vi "Set_Gain_DHPCA-100.vi"(3 "error in":errorcluster, 4 "Status":i32, 5 "Gain  [V/A]":T1(ring), 6 "index":i32) -> (0 "error out":errorcluster, 1 "Status_out":i32, 2 "index_out":i32)   [LabVIEW 2010, in "FEMTO_LUCI-10.lvlib"]
uses:
  <userlib>/FEMTO/FEMTO_LUCI-10.lvlib
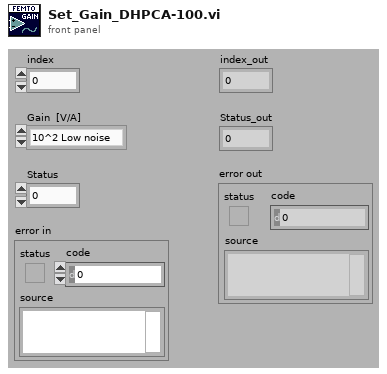
[diagram p1: front panel]
types:
  T1 = enum16{"10^2 Low noise", "10^3 Low noise", "10^4 Low noise", "10^5 Low noise", "10^6 Low noise", "10^7 Low noise", "10^3 High speed", "10^4 High speed", "10^5 High speed", "10^6 High speed", "10^7 High speed", "10^8 High speed"}
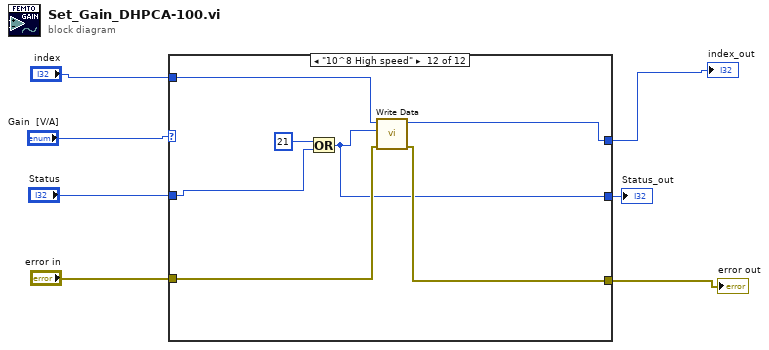
[diagram p0: block diagram]
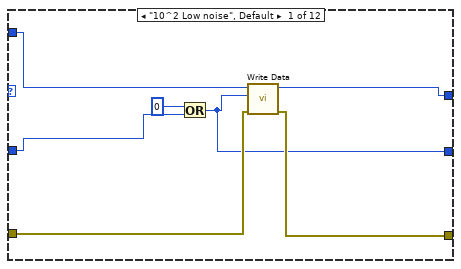
[diagram p2: hidden frame]
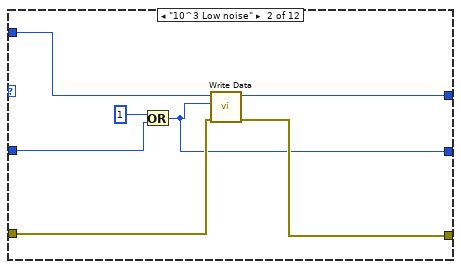
[diagram p3: hidden frame]
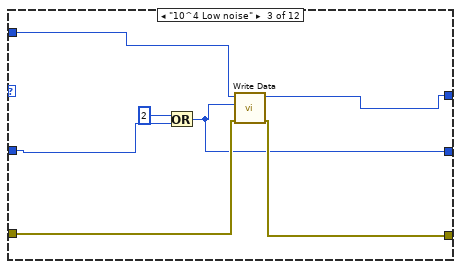
[diagram p4: hidden frame]
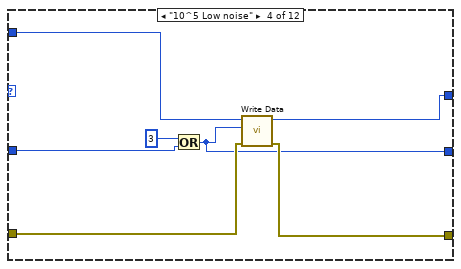
[diagram p5: hidden frame]
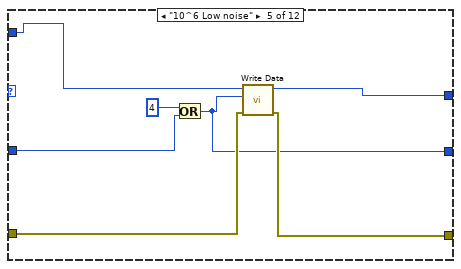
[diagram p6: hidden frame]
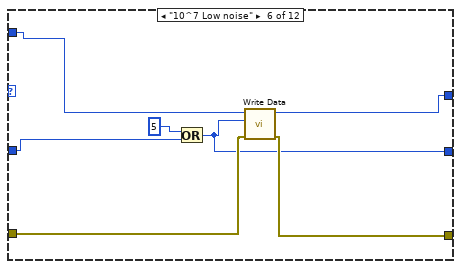
[diagram p7: hidden frame]
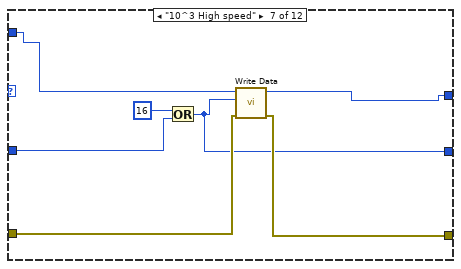
[diagram p8: hidden frame]
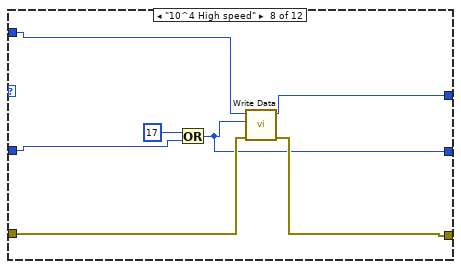
[diagram p9: hidden frame]
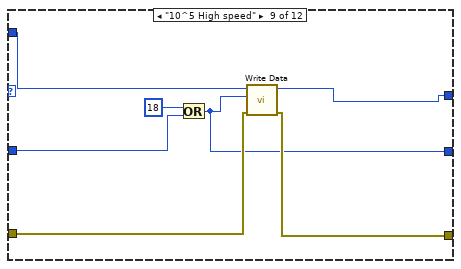
[diagram p10: hidden frame]
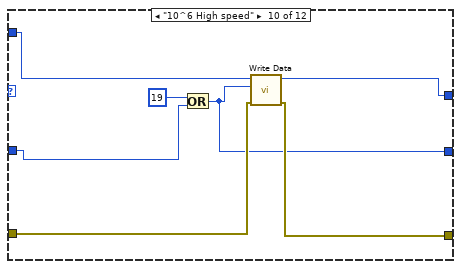
[diagram p11: hidden frame]
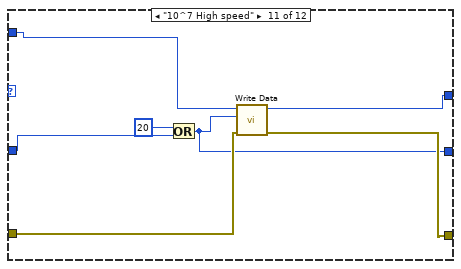
[diagram p12: hidden frame]
diagram:
  n1 = case shown="\"10^8 High speed\"" "Gain  [V/A]" {
    tunnel: "index" -> [w12 w21 w26 w33 w41 w48 w55 w61 w68 w76 w82 w89]
    tunnel: [w11 w20 w25 w32 w40 w47 w54 w62 w69 w75 w83 w88] -> w2
    tunnel: "error in" -> [w9 w19 w23 w30 w38 w45 w52 w60 w66 w73 w80 w86]
    tunnel: [w10 w18 w24 w31 w39 w46 w53 w59 w67 w74 w79 w87] -> w4
    tunnel: "Status" -> [w13 w17 w27 w34 w37 w44 w51 w58 w65 w72 w81 w90]
    tunnel: [w8 w15 w22 w29 w36 w43 w50 w57 w64 w71 w78 w85] -> w7
    frame "10^2 Low noise", Default {
      n2 = Or(x=0 ("data_low"), y=w13) -> (x .or. y?=w8:i32)
      n3 = call <userlib>:"Write Data.vi"("error in (no error)"=w9, "data_low"=w8, "index"=w12) -> ("error out"=w10:errorcluster, "index_out"=w11:i32)  [unwired: 1 in, 6 out]
    }
    frame "10^3 Low noise" {
      n4 = Or(x=1 ("data_low"), y=w17) -> (x .or. y?=w15:i32)
      n5 = call <userlib>:"Write Data.vi"("error in (no error)"=w19, "data_low"=w15, "index"=w21) -> ("error out"=w18:errorcluster, "index_out"=w20:i32)  [unwired: 1 in, 6 out]
    }
    frame "10^4 Low noise" {
      n6 = Or(x=2 ("data_low"), y=w27) -> (x .or. y?=w22:i32)
      n7 = call <userlib>:"Write Data.vi"("error in (no error)"=w23, "data_low"=w22, "index"=w26) -> ("error out"=w24:errorcluster, "index_out"=w25:i32)  [unwired: 1 in, 6 out]
    }
    frame "10^5 Low noise" {
      n8 = Or(x=3 ("data_low"), y=w34) -> (x .or. y?=w29:i32)
      n9 = call <userlib>:"Write Data.vi"("error in (no error)"=w30, "data_low"=w29, "index"=w33) -> ("error out"=w31:errorcluster, "index_out"=w32:i32)  [unwired: 1 in, 6 out]
    }
    frame "10^6 Low noise" {
      n10 = Or(x=4 ("data_low"), y=w37) -> (x .or. y?=w36:i32)
      n11 = call <userlib>:"Write Data.vi"("error in (no error)"=w38, "data_low"=w36, "index"=w41) -> ("error out"=w39:errorcluster, "index_out"=w40:i32)  [unwired: 1 in, 6 out]
    }
    frame "10^7 Low noise" {
      n12 = Or(x=5 ("data_low"), y=w44) -> (x .or. y?=w43:i32)
      n13 = call <userlib>:"Write Data.vi"("error in (no error)"=w45, "data_low"=w43, "index"=w48) -> ("error out"=w46:errorcluster, "index_out"=w47:i32)  [unwired: 1 in, 6 out]
    }
    frame "10^3 High speed" {
      n14 = Or(x=16 ("data_low"), y=w51) -> (x .or. y?=w50:i32)
      n15 = call <userlib>:"Write Data.vi"("error in (no error)"=w52, "data_low"=w50, "index"=w55) -> ("error out"=w53:errorcluster, "index_out"=w54:i32)  [unwired: 1 in, 6 out]
    }
    frame "10^4 High speed" {
      n16 = Or(x=17 ("data_low"), y=w58) -> (x .or. y?=w57:i32)
      n17 = call <userlib>:"Write Data.vi"("error in (no error)"=w60, "data_low"=w57, "index"=w61) -> ("error out"=w59:errorcluster, "index_out"=w62:i32)  [unwired: 1 in, 6 out]
    }
    frame "10^5 High speed" {
      n18 = Or(x=18 ("data_low"), y=w65) -> (x .or. y?=w64:i32)
      n19 = call <userlib>:"Write Data.vi"("error in (no error)"=w66, "data_low"=w64, "index"=w68) -> ("error out"=w67:errorcluster, "index_out"=w69:i32)  [unwired: 1 in, 6 out]
    }
    frame "10^6 High speed" {
      n20 = Or(x=19 ("data_low"), y=w72) -> (x .or. y?=w71:i32)
      n21 = call <userlib>:"Write Data.vi"("error in (no error)"=w73, "data_low"=w71, "index"=w76) -> ("error out"=w74:errorcluster, "index_out"=w75:i32)  [unwired: 1 in, 6 out]
    }
    frame "10^7 High speed" {
      n22 = Or(x=20 ("data_low"), y=w81) -> (x .or. y?=w78:i32)
      n23 = call <userlib>:"Write Data.vi"("error in (no error)"=w80, "data_low"=w78, "index"=w82) -> ("error out"=w79:errorcluster, "index_out"=w83:i32)  [unwired: 1 in, 6 out]
    }
    frame "10^8 High speed" {
      n24 = Or(x=21 ("data_low"), y=w90) -> (x .or. y?=w85:i32)
      n25 = call <userlib>:"Write Data.vi"("error in (no error)"=w86, "data_low"=w85, "index"=w89) -> ("error out"=w87:errorcluster, "index_out"=w88:i32)  [unwired: 1 in, 6 out]
    }
  }
  "index_out" <- w2
  "error out" <- w4
  "Status_out" <- w7
